vi "WriteFile.vi"(6 "Overwrite?(F)":bool, 8 "error in (no error)":errorcluster, 9 "Proposed File Name":string, 10 "Output Path":path, 11 "CarexData In":refnum<class "ExpData.lvclass">) -> (0 "error out":errorcluster, 1 "Actual File Name":string, 3 "CarexData Out":refnum<class "ExpData.lvclass">)   [LabVIEW 2016, in "ExpData.lvclass"]
uses:
  ExpData.lvclass
  ExpData.lvclass/ExpData.ctl
  <vilib>/Utility/file.llb/Write Delimited Spreadsheet (DBL).vi
  <vilib>/GoldZinc Software/auzn custom VIs/CustomVI.lvlib
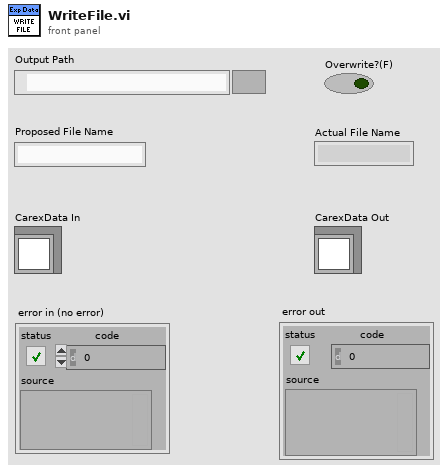
[diagram p1: front panel]
types:
  T1 = enum16{"Native", "Native Command Line", "UNIX", "Macintosh", "DOS"}
  T2 = enum16{"open", "replace", "create", "open or create", "replace or create", "replace or create with confirmation"}
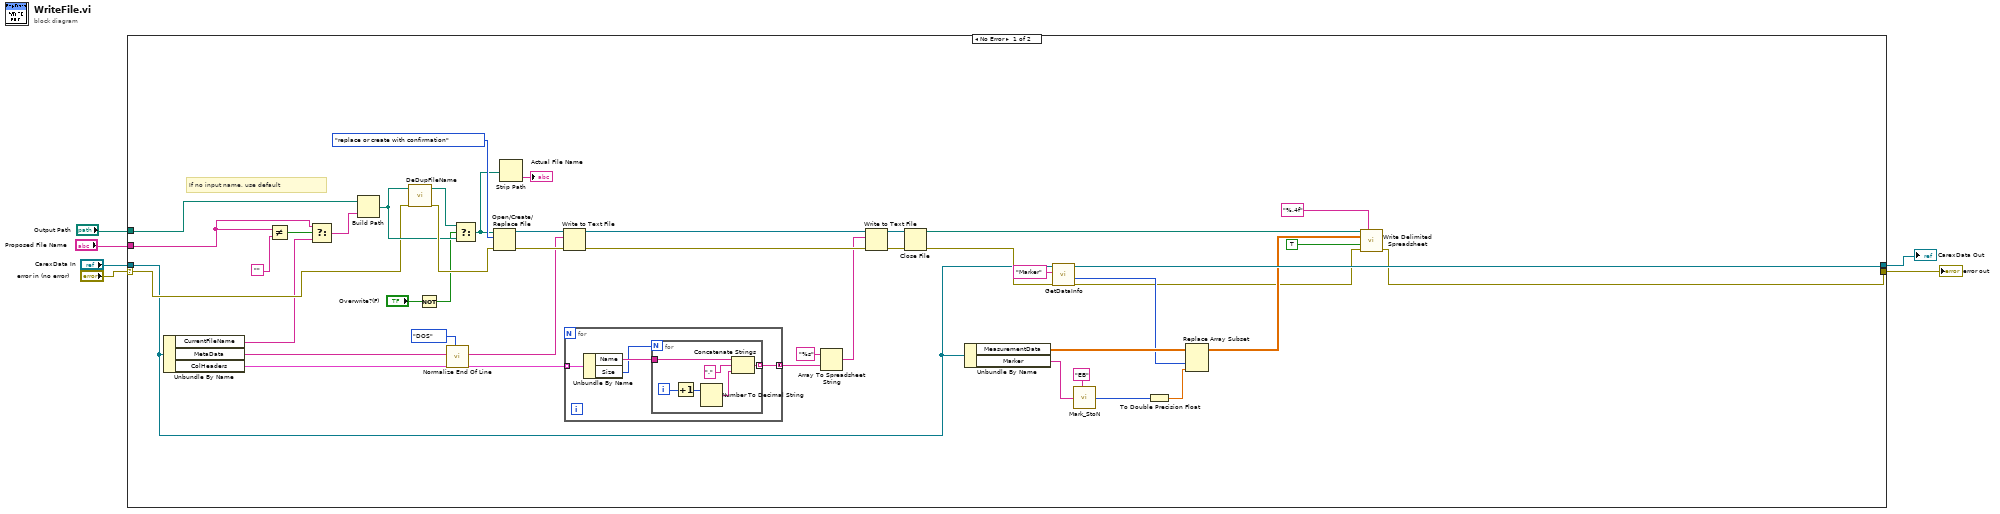
[diagram p0: block diagram]
diagram:
  n1 = case shown="No Error" "error in (no error)" {
    selector: "error in (no error)" -> [w36 w62]
    tunnel: [w25 w61] -> w5
    tunnel: [w7 w62] -> w6
    tunnel: "Output Path" -> [w44 _]
    tunnel: "CarexData In" -> [w16 w61]
    tunnel: "Proposed File Name" -> [w48 _]
    frame No Error {
      # "If no input name, use default"
      n2 = Unbundle By Name(w16) -> ("CurrentFileName"=w15:string, "MetaData"=w13:string, "ColHeaders"=w14:cluster{"Name":string, "Index":i8, "Size":i8}[])
      n3 = Not Equal?(x=w48, y="") -> (x != y?=w49:bool)
      n4 = Select(t=w48, s=w49, f=w15) -> (s? t:f=w43:string)
      n5 = Build Path(base path=w44, name or relative path=w43) -> (appended path=w41:path)
      n6 = call <vilib>:"DeDupFileName.vi"("error in (no error)"=w36, "Path"=w41) -> ("error out"=w42:errorcluster, "Out Path"=w47:path)  [unwired: 7 in, 1 out]
      n7 = Not(x="Overwrite?(F)") -> (.not. x?=w40:bool)
      n8 = call <vilib>:"Normalize End Of Line.vi"("end of line (Native)"=T1."DOS", "string in"=w13) -> ("string out"=w12:string)  [unwired: 6 in]
      n9 = Select(t=w47, s=w40, f=w41) -> (s? t:f=w39:path)
      n10 = Open/Create/Replace File(file path (use dialog)=w39, error in=w42, operation (0:open)=T2."replace or create with confirmation") -> (refnum out=w18:refnum<file>, error out=w17:errorcluster)  [unwired: 3 in, 1 out]
      n11 = Strip Path(path=w39) -> (name=→"Actual File Name":string)  [unwired: 1 out]
      n12 = Write to Text File(file (use dialog)=w18, text=w12, error in=w17) -> (refnum out=w35:refnum<file>, error out=w34:errorcluster)  [unwired: 1 in, 1 out]
      n13 = for {
        tunnel: w14 -> [w54] mode=indexing
        tunnel: [w51] -> w31 mode=concatenating
        n14 = Unbundle By Name(w54) -> ("Name"=w53:string, "Size"=w52:i8)
        n15 = for {
          N: w52 -> [_]
          tunnel: w53 -> [w57]
          tunnel: [w55] -> w51 mode=indexing
          i -> [w60]
          n16 = Increment(x=w60) -> (x+1=w59:i32)
          n17 = Number To Decimal String(number=w59) -> (decimal integer string=w58:string)  [unwired: 1 in]
          n18 = Concatenate Strings(w57, "." ("format string"), w58) -> (w55:string)
        }
      }
      n19 = Array To Spreadsheet String(array=w31, 3:"%s" ("format string")) -> (spreadsheet string=w29:string)  [unwired: 1 in]
      n20 = Write to Text File(file (use dialog)=w35, text=w29, error in=w34) -> (refnum out=w33:refnum<file>, error out=w32:errorcluster)  [unwired: 1 in, 1 out]
      n21 = Close File(refnum=w33, error in=w32) -> (path=w37:path, error out=w24:errorcluster)
      n22 = Unbundle By Name(w16) -> ("MeasurementData"=w22:dbl[][], "Marker"=w26:string[])
      n23 = call "GetDataInfo.vi"("error in (no error)"=w24, "Name"="Marker", "CarexMData in"=w16) -> ("error out"=w8:errorcluster, "Index"=w10:i8, "CarexMData out"=w25:refnum<class "ExpData.lvclass">)  [unwired: 4 in, 2 out]
      n24 = call "Mark_StoN.vi"("Marker(Low->High)"="EB", "MarkerString"=w26) -> ("MarkerNumber"=w21:u32[])  [unwired: 3 in]
      n25 = To Double Precision Float(number=w21) -> (double precision float=w20:dbl[])
      n26 = Replace Array Subset(array=w22, new element=w20, index (col)=w10) -> (w19:dbl[][])  [unwired: 1 in]
      n27 = call-poly <vilib>:"Write Delimited Spreadsheet.vi"("file path (dialog if empty)"=w37, "format (%.3f)"="%.4f", "2D data"=w19, "append to file? (new file:F)"=TRUE, "error in (no error)"=w8) -> ("error out"=w7:errorcluster)  [unwired: 9 in, 1 out]
    }
    frame Error {
    }
  }
  "CarexData Out" <- w5
  "error out" <- w6
